vi "Fetch Single Point From Load.vi"(8 "error in (no error)":errorcluster, 11 "Reference values":T1={"dcpower session reservation"=refnum, "Source handle array"=[], "Source channel name array"=[], "Load handle"="", "Load channel name"="", "Source voltage values"=[], "Load current values"=[], "Number of steps"=0, "Source sequence name"="", "Source terminal name"="", "Measure terminal name"="", "scope session reservation"=refnum, "Scope handles"=[], "connection map"={}, "instrument info map array"=[], "Enable TClk"=FALSE, "dmm session reservation"=refnum, "dmm handle array"=[], "DMM Trigger Source"=enum."Immediate", "DMM Sample Trigger"=enum."TTL 0", "Measurement Results"={"Status"="", "Voltage values"=[], "Source sweep points"=0, "Load sweep points"=0, "Source voltages"=[], "Source currents"=[], "Load voltages"=[], "Load currents"=[], "Load voltage deviation"=[], "Efficiency"=[], "Maximum efficiency"=[], "Minimum load voltage"=[], "Maximum load voltage"=[], "Minimum load regulation"=[], "Maximum load regulation"=[], "waveform pins"=[], "waveform sites"=[], "waveform t0 array"=[], "waveform dt array"=[], "waveform length array"=[], "concatenated waveform Y"=[]}, "Additional measurements"={"voltage measurements from all sources"=[], "current measurements from all sources"=[], "all dmm measurements"=[], "all scope waverforms"=[]}}) -> (0 "error out":errorcluster, 1 "current measurements":dbl[](array[numeric]), 2 "voltage measurements":dbl[](array[numeric]), 3 "Reference values out":T1={"dcpower session reservation"=refnum, "Source handle array"=[], "Source channel name array"=[], "Load handle"="", "Load channel name"="", "Source voltage values"=[], "Load current values"=[], "Number of steps"=0, "Source sequence name"="", "Source terminal name"="", "Measure terminal name"="", "scope session reservation"=refnum, "Scope handles"=[], "connection map"={}, "instrument info map array"=[], "Enable TClk"=FALSE, "dmm session reservation"=refnum, "dmm handle array"=[], "DMM Trigger Source"=enum."Immediate", "DMM Sample Trigger"=enum."TTL 0", "Measurement Results"={"Status"="", "Voltage values"=[], "Source sweep points"=0, "Load sweep points"=0, "Source voltages"=[], "Source currents"=[], "Load voltages"=[], "Load currents"=[], "Load voltage deviation"=[], "Efficiency"=[], "Maximum efficiency"=[], "Minimum load voltage"=[], "Maximum load voltage"=[], "Minimum load regulation"=[], "Maximum load regulation"=[], "waveform pins"=[], "waveform sites"=[], "waveform t0 array"=[], "waveform dt array"=[], "waveform length array"=[], "concatenated waveform Y"=[]}, "Additional measurements"={"voltage measurements from all sources"=[], "current measurements from all sources"=[], "all dmm measurements"=[], "all scope waverforms"=[]}})   [LabVIEW 2021, in "Efficiency And Load Regulation with Pin Map.lvlib"]
uses:
  Efficiency And Load Regulation with Pin Map.lvlib
  Reference values.ctl
  <vilib>/Plug-In SDKs/Clients/Session Management V1/Session Reservation/Session Reservation.lvclass
  common/Instrument Control/Scope/TClk/Instrument Info.ctl
  common/Instrument Control/Scope Parameters.ctl
  <instrlib>/niScope/Controls/niScope vertical coupling.ctl
  <instrlib>/niDMM/nidmm.llb/niDMM Trigger.ctl
  <instrlib>/niDMM/nidmm.llb/niDMM Sample Trigger.ctl
  Measurement Results.ctl
  Additional measurements.ctl
  common/PMIC Common.lvlib
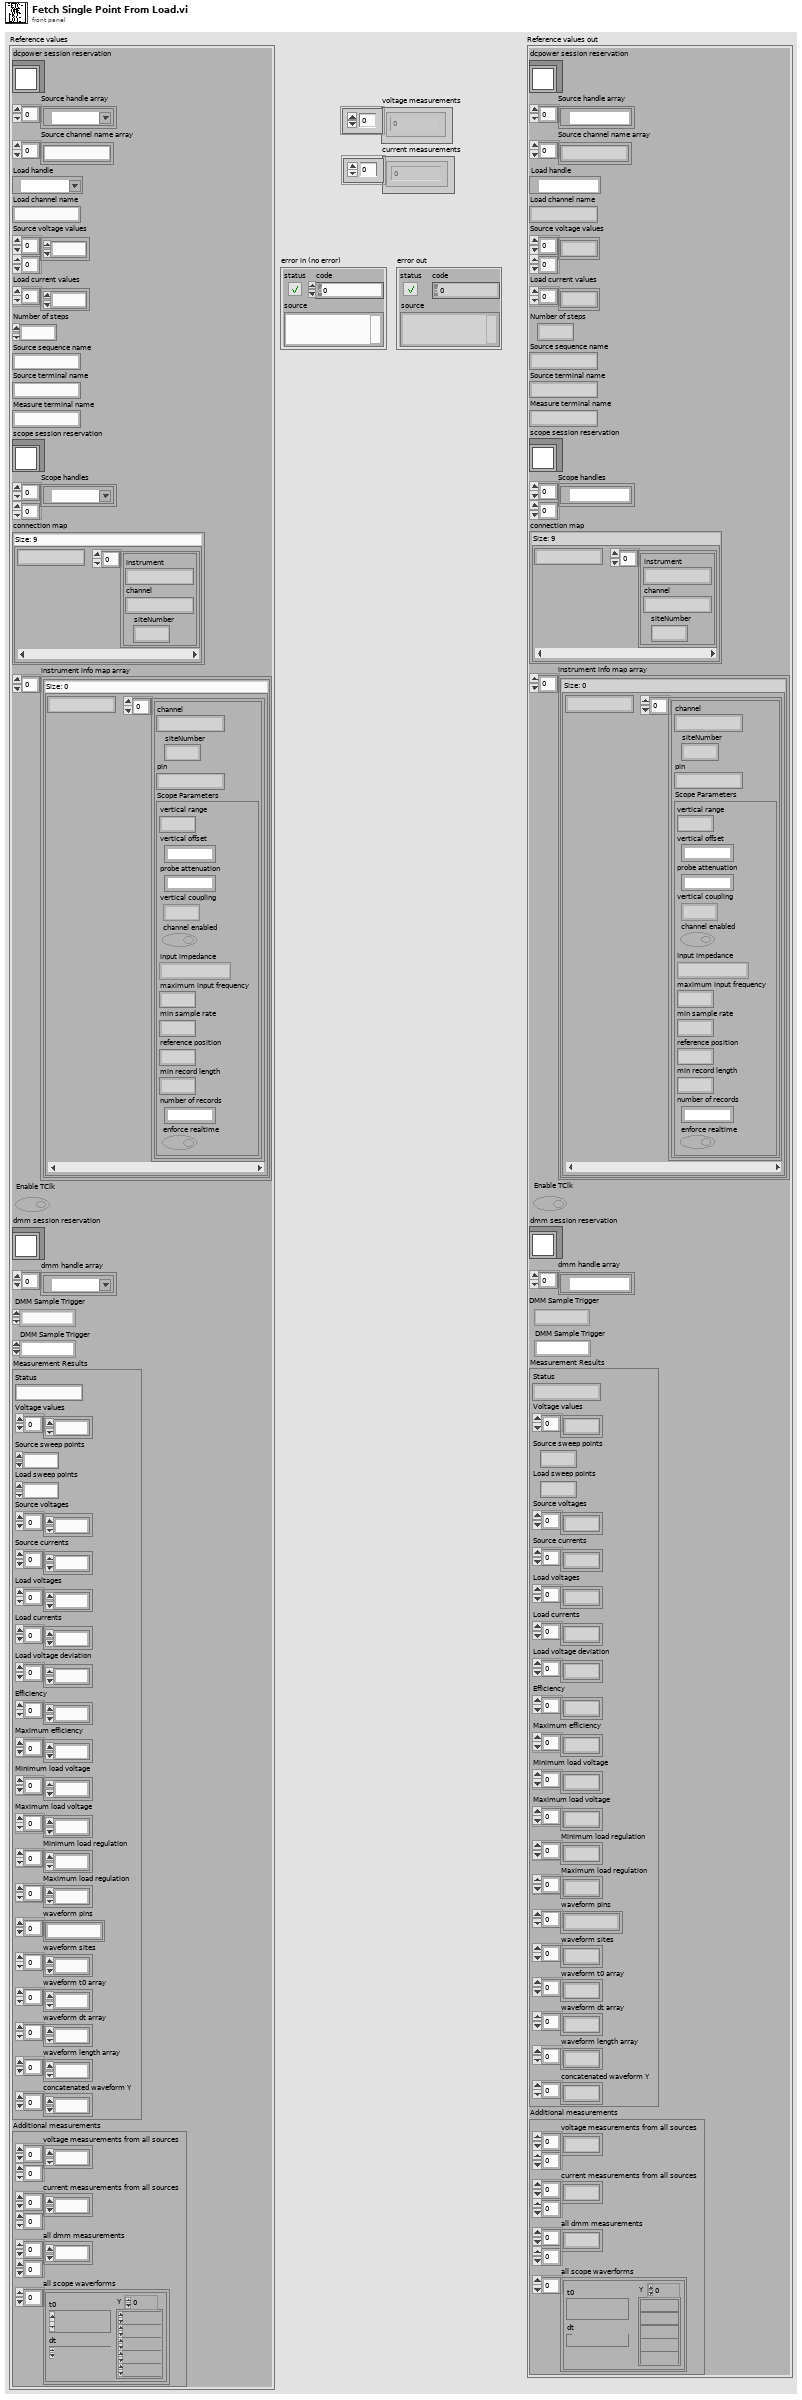
[diagram p1: front panel]
types:
  T1 = typedef "Efficiency And Load Regulation with Pin Map.lvlib/Reference values.ctl" = cluster{"dcpower session reservation":refnum<class "Session Reservation.lvclass">, "Source handle array":refnum<k15>[], "Source channel name array":string[], "Load handle":refnum<k15>, "Load channel name":string, "Source voltage values":dbl[][], "Load current values":dbl[], "Number of steps":i32, "Source sequence name":string, "Source terminal name":string, "Measure terminal name":string, "scope session reservation":refnum<class "Session Reservation.lvclass">, "Scope handles":refnum<k15>[][], "connection map":map{string, T2[]}, "instrument info map array":map{string, cluster{"channel":string, "siteNumber":i32, "pin":string, "Scope Parameters":T3}[]}[], "Enable TClk":bool, "dmm session reservation":refnum<class "Session Reservation.lvclass">, "dmm handle array":refnum<k15>[], "DMM Trigger Source":T5, "DMM Sample Trigger":T6, "Measurement Results":T7, "Additional measurements":T8}
  T2 = typedef "PMIC Common.lvlib/Instrument Info.ctl" = cluster{"instrument":string, "channel":string, "siteNumber":i32}
  T3 = typedef "PMIC Common.lvlib/Scope Parameters.ctl" = cluster{"vertical range":dbl, "vertical offset":dbl, "probe attenuation":dbl, "vertical coupling":T4, "channel enabled":bool, "input impedance":u32, "maximum input frequency":dbl, "min sample rate":dbl, "reference position":dbl, "min record length":i32, "number of records":i32, "enforce realtime":bool}
  T4 = typedef "niScope vertical coupling.ctl" = i32
  T5 = typedef "niDMM Trigger.ctl" = enum16{"Immediate", "External", "TTL 0", "TTL 1", "TTL 2", "TTL 3", "TTL 4", "TTL 5", "TTL 6", "Software", "TTL 7", "PXI Star", "LBR Trig 1", "Aux Trig 1"}
  T6 = typedef "niDMM Sample Trigger.ctl" = enum16{"Immediate", "External", "TTL 0", "TTL 1", "TTL 2", "TTL 3", "TTL 4", "TTL 5", "TTL 6", "Interval", "Software", "TTL 7", "PXI Star", "LBR Trig 1", "Aux Trig 1"}
  T7 = typedef "Efficiency And Load Regulation with Pin Map.lvlib/Measurement Results.ctl" = cluster{"Status":string, "Voltage values":dbl[], "Source sweep points":i32, "Load sweep points":i32, "Source voltages":dbl[], "Source currents":dbl[], "Load voltages":dbl[], "Load currents":dbl[], "Load voltage deviation":dbl[], "Efficiency":dbl[], "Maximum efficiency":dbl[], "Minimum load voltage":dbl[], "Maximum load voltage":dbl[], "Minimum load regulation":dbl[], "Maximum load regulation":dbl[], "waveform pins":string[], "waveform sites":i32[], "waveform t0 array":dbl[], "waveform dt array":dbl[], "waveform length array":i32[], "concatenated waveform Y":dbl[]}
  T8 = typedef "Efficiency And Load Regulation with Pin Map.lvlib/Additional measurements.ctl" = cluster{"voltage measurements from all sources":dbl[][], "current measurements from all sources":dbl[][], "all dmm measurements":dbl[][], "all scope waverforms":waveform(dbl)[]}
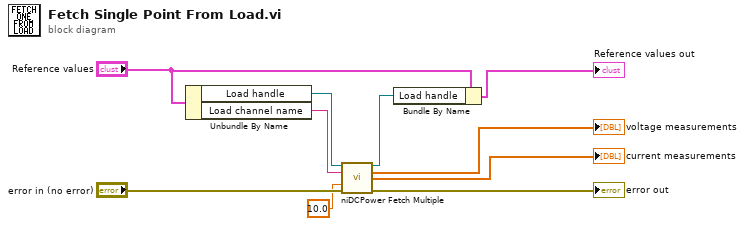
[diagram p0: block diagram]
diagram:
  n1 = Unbundle By Name("Reference values") -> ("Load handle"=w10:refnum<k15>, "Load channel name"=w9:string)
  n2 = call <instrlib>:"niDCPower Fetch Multiple.vi"("instrument handle"=w10, "channel name"=w9, "timeout (1.0)"=10.0, "error in (no error)"="error in (no error)") -> ("instrument handle out"=w5:refnum<k15>, "voltage measurements"=→"voltage measurements":dbl[], "current measurements"=→"current measurements":dbl[], "error out"=→"error out":errorcluster)  [unwired: 1 in, 7 out]
  n3 = Bundle By Name(cluster="Reference values", "Load handle"=w5) -> (→"Reference values out":T1)
